vi "Standardabweichung und Varianz.vi"(9 "Gewichtung (Stichprobe)":T1, 11 "X":sgl[](array[numeric]) format="%.2f") -> (0 "Varianz":sgl format="%.2f", 2 "Mittelwert":sgl format="%.2f", 3 "Standardabweichung":sgl format="%.2f")   [LabVIEW 2020, in "Messdaten.lvlib"]
uses:
  Messdaten.lvlib
  Gewichtung (Stichprobe).ctl
panel:
  # "Standardabweichung und Varianz"
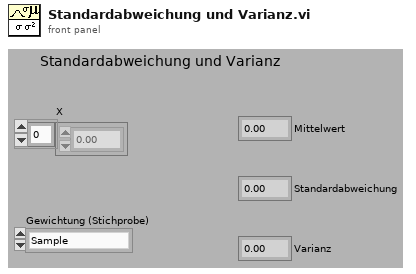
[diagram p1: front panel]
types:
  T1 = typedef "Messdaten.lvlib/Gewichtung (Stichprobe).ctl" = enum16{"Sample", "Population"}
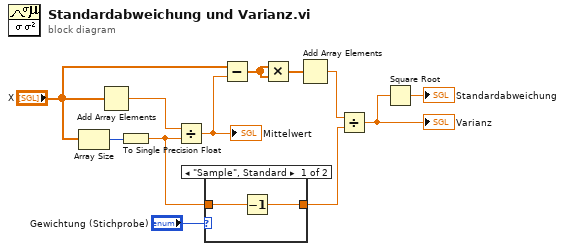
[diagram p0: block diagram]
diagram:
  n1 = Array Size(array="X") -> (size(s)=w12:i32)
  n2 = Add Array Elements(numeric array="X") -> (sum=w11:sgl)
  n3 = To Single Precision Float(number=w12) -> (single precision float=w5:sgl)
  n4 = Divide(x=w11, y=w5) -> (x/y=w9:sgl)
  "Mittelwert" <- w9
  n5 = case shown="\"Sample\", Standard" "Gewichtung (Stichprobe)" {
    tunnel: w5 -> [w14 w15]
    tunnel: [w13 w15] -> w3
    frame "Sample", Default {
      n6 = Decrement(x=w14) -> (x-1=w13:sgl)
    }
    frame "Population" {
    }
  }
  n7 = Subtract(x="X", y=w9) -> (x-y=w8:sgl[])
  n8 = Multiply(x=w8, y=w8) -> (x*y=w7:sgl[])
  n9 = Add Array Elements(numeric array=w7) -> (sum=w4:sgl)
  n10 = Divide(x=w4, y=w3) -> (x/y=w2:sgl)
  "Varianz" <- w2
  n11 = Square Root(x=w2) -> (sqrt(x)=→"Standardabweichung":sgl)
